vi "create.vi"(8 "error in (no error)":errorcluster) -> (0 "error out":errorcluster, 3 "tree (dvr)":refnum<data-value>)   [LabVIEW 2015, in "binary_tree.lvlib"]
uses:
  binary_tree.lvlib
  _Controls/tree.ctl
  _Controls/node_key.ctl
  _Controls/node_data.ctl
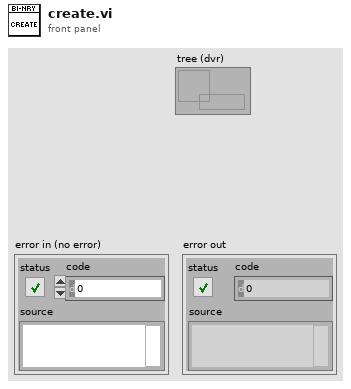
[diagram p1: front panel]
types:
  T1 = typedef "binary_tree.lvlib/tree.ctl" = cluster{"key":T2, "data":T3, "node_dvr (left)":variant, "node_dvr (right)":variant}
  T2 = typedef "binary_tree.lvlib/node_key.ctl" = cluster{dbl}
  T3 = typedef "binary_tree.lvlib/node_data.ctl" = cluster{dbl}
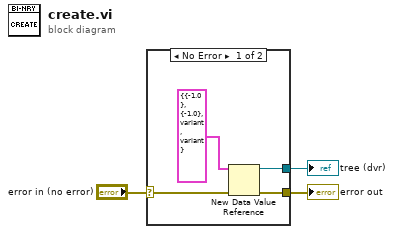
[diagram p0: block diagram]
diagram:
  n1 = case shown="No Error" "error in (no error)" {
    selector: "error in (no error)" -> [w7 w8]
    tunnel: [w6 w8] -> w2
    tunnel: [w5 _] -> w1
    frame No Error {
      n2 = New Data Value Reference(data value=T1 {"key"={-1.0}, "data"={-1.0}, "node_dvr (left)"=variant, "node_dvr (right)"=variant} ("Node out"), error in=w7) -> (data value reference=w5:refnum<data-value>, error out=w6:errorcluster)
    }
    frame Error {
    }
  }
  "error out" <- w2
  "tree (dvr)" <- w1
